vi "Bingo Lose.vi"() -> ()   [LabVIEW 2020]
uses:
  <vilib>/regexp/Match Regular Expression.xnode
panel:
  out "Losing Board":cluster{i32, bool}[][](array[cluster])
  out "x*y":i32
  out "Picks":string
  in  "Input":string="46,12,57,37,14,78,31,71,87,52,64,97,10,35,54,36,27,84,80,94,99,22,0,11,30,44,86,59,66,7,90,21,51,53,92,8,76,41,39,77,42,88,29,24,60,17,68,13,79,67,50,82,25,61,20,16,6,3,81,19,85,9,28,56,75,96,2,26,1,62,33,63,32,73,18,48,43,65,98,5,91,69,47,4,38,23,49,34,55,83,93,45,72,95,40,15,58,74,70,89\n\n37 72 60 35 89\n32 49  4 77 82\n30 26 27 63 88\n29 43 16 34 58\n48 33 96 79 94\n\n41 94 77 43 87\n 2 17 82 96 25\n95 49 32 12  9\n59 33 67 71 64\n88 54 93 85 30\n\n78 84 73 64 81\n 6 66 54 21 15\n72 88 69  5 93\n11 96 38 95 44\n13 41 94 55 48\n\n 5 14  2 82 33\n56 26  0 84 92\n 8 95 24 54 25\n68 67 15 85 47\n20 91 36 13 88\n\n39 26 33 65 32\n78 72 80 51  0\n35 64 60 18 31\n93 59 83 54 74\n86  5  9 98 69\n\n 0  8 20 18 70\n 5 29 65 21 57\n68 61 83 63 51\n91 73 77 75 80\n35 62 16 32 10\n\n51 78 58 67 93\n50 14 99  5 31\n 6 21 48 30 83\n22 33 23  1 34\n 2 72 57 54 42\n\n15 68  4 24 49\n12  9 74 88 51\n91 19 50 76 75\n80 84 23 17 53\n67 42 22 85 36\n\n41 78 11 69  9\n90 25 98 65 77\n97 53 37 84 89\n58 63  5 55  1\n24 10 74 20 82\n\n42 19 95 89 49\n61 31 50 76  3\n34 47 32 69 86\n78 68 99 11 91\n55 12 73 45 23\n\n24 53 95 64 14\n40 29 71 57 97\n62 70 25 22  2\n88 68 33 82 59\n72 38 76 78 43\n\n73 36 84 90 40\n16  4 57  9 29\n38 97 46 51 83\n86 88 99 44 32\n54 49 37 43 62\n\n18 66 17 49 27\n24 93 91 87 72\n54 37 77 43 10\n88 80 60 15 79\n47 68 12  2 69\n\n 9 23 13 57 68\n38 97 63 88 98\n96 62 65 82 58\n61 83 29 47 40\n21 86 20 16 56\n\n27 90 37 97 52\n14 96 76 21 79\n 0 43 63 81 56\n42 62 23 55 74\n45 72 77 44 47\n\n 8 78 63 24 87\n 9 23 12 17 68\n36 83 45 61 50\n84 77 18 86 37\n31 26 19 49 94\n\n72 84 59 48 40\n92 98 35  1 80\n83 15 85 63 39\n 2 64 58 13 20\n29 88 60 12 74\n\n21 94 52  6  4\n89 70 39 23 64\n96 87 31 54 14\n88 35 83 13 56\n84 10 98 48 68\n\n70 33 48 21 37\n91 95 65 38 77\n92 14 26 96 60\n12  6 73 13 81\n54 55  2 45 80\n\n60 11 67 95 28\n 5 32  0 71 12\n47 78 13 54 43\n49 89 82 66 77\n26 53 19 79  3\n\n81  9 53 72 29\n56 35 60 44 45\n42 94 96 88 64\n15 92  4  6 14\n97 11 17 61 63\n\n24 43 33  9 34\n36 28 69 35  7\n47  4 14 82 38\n11  1 52  0 49\n93 87 98 41  5\n\n37 79 99 34 77\n38 26 25 95 70\n28 78 40 33 86\n41 57 96 10 24\n 9 74 72 50 81\n\n18 96 52 29 61\n38 90  1 48 51\n78 11 27 55 97\n33 21 87 93 67\n79 46 94 45  2\n\n27 63  6 90 10\n 3 60 24  5 89\n78 72 76 54  8\n33 22 87 51 58\n 4 37 64 91 43\n\n63 73 87 80 89\n29 14 95 48  3\n71 55 69  9 67\n30 99 19  2 86\n26 72 88 85 37\n\n12 57 81 78 40\n35  4 55 15 39\n33 45 25 60 70\n86 79 88 52  3\n90 20 28 59 85\n\n92 51 98 47 99\n41 78 65  4 46\n19 87 39 89 17\n12 23 36 29 44\n 6 82 71 16 37\n\n 8 34 81 67 80\n83 92 13 11 41\n39 89 93 49 43\n20 69  3 74 76\n44 72 68 70 45\n\n66 39 94 98 28\n72  4 25 77 76\n56 41 84 59 40\n36 87 18 44 73\n29 45 79 55 95\n\n45 91  2 92 16\n21 47 86 81 56\n31 11 62  5 95\n39  1 30 65 33\n42 60 17 18 83\n\n86 11 77 30 43\n51 88 73 98 94\n72 63 38 56 10\n57 92 49  7 41\n79 75 34 23 54\n\n56 95  3 43 65\n39 62 93 19 27\n61 41 99 96 52\n 4 92 77 98 70\n16 54 11 17 57\n\n 6 63 10 71 58\n64 70 50 92  0\n 7 14 99 45 26\n78 17 44 46 73\n77 38 62 53 37\n\n31 82 67 55 27\n57 58 84  6 15\n14 41 49  8 85\n12 32 91 42 19\n23  1 87 54 29\n\n54 60 43 26  4\n78 17 28 67  5\n87 93 90 71 22\n13 30 16 21 85\n55 74 52  1 29\n\n50 16 70 32 33\n 6 94 52 66 22\n97 64 98 72 39\n27 69 99 34 26\n36 91 37 21 14\n\n 7 97 64 28 18\n85 80 14 37 34\n72  1 22 58 73\n53  3 68 17  0\n29 44 56 95 32\n\n30 66 93 24 92\n48 80 79 86 27\n89 13 62 94 81\n70 65 61  8 54\n96 97 20 90 34\n\n87 76  4  7 43\n92 55 80 25 62\n79  6 88 35 30\n10 32  5 45 17\n36 27 33 68 63\n\n72 69 27 88 41\n34 53 42 84  3\n58 18 22 66 65\n 9 47 85 12 62\n73 90 91 57 33\n\n67 16 50 58 52\n68 70 84 98 69\n 4 72  9 64  0\n93 97 39 26  5\n 3 37 79  7 82\n\n61 57 88 54 70\n77  8 94 81 63\n39 48 18 13 10\n55 23 27  4 73\n 3  5 64  0 96\n\n62 27  0 52 19\n28 57 83 25 41\n 5 59 24 33 80\n37 85  2 86 43\n22 94 50  8 20\n\n54 32 34 47 87\n71 22 43 85 24\n11 68 58 36 46\n35 56 61 67 18\n70 23 72  5 59\n\n 3 96 41 45 32\n68  2 56 28 24\n87 38 40 75 26\n53 64 73 80 81\n54 88 20  6 18\n\n64 55 51 96 47\n59 35 49 67 71\n36 91 61 76 68\n 6 94 20  8 27\n60 88 45  7 82\n\n87 94 51 91  1\n96 60 28 97 37\n26 27 74 53 35\n88 89 11 77  8\n73 47 18 59  6\n\n46 50 19 36 83\n69 28  4 44 70\n45 20 63 27  1\n53 38  9 47 67\n91 31 79 73 86\n\n45  3 98 91 60\n40  7 78 34 83\n52 73 59 13  4\n38 15 82 86 79\n42 11 17 20 62\n\n65 86 38 20 72\n78 45 73 74 25\n62 42 24 75  3\n81  8 35 50 51\n44 11 94 85 57\n\n13 86 55 65 96\n53 18 43 76 20\n41 14 32 52 38\n90 59 80 68  7\n 2 23 92 39 50\n\n96 62 85 24 14\n37  5 11 91 45\n61 28 23 34 77\n43 48 20  0 21\n10 35  2 26 97\n\n89  5 40 34 84\n90  6 72 68 10\n13 64 71 31 76\n53 60  9 92 62\n69 98  8 50  3\n\n17 86 10 75 79\n67 94 78 40 56\n11 85 82 50 46\n53 39 22  9 61\n59 73 72 33 45\n\n65 22 18 96 95\n55 86 67 52 69\n10  2 60 83 98\n43 61 87 88 66\n41 24  8 84 33\n\n31 53 98 70 91\n33 34 48 83  9\n40 39 29 71 65\n69 10 62 30  4\n52 21 11 93 75\n\n 8 94 53 85 89\n13 84 58 59 29\n97  7 21 25 96\n45 54 34 22 63\n37 17 49 68 67\n\n86 87 84 24 10\n82 32 36 59 50\n 8 62 79 71 43\n49 23 85 69 58\n21 66 42 25 56\n\n65 88 43 25 19\n26 36 63  5  6\n37 54 75  1 38\n95 46 83 66 28\n 4 90 80 99 85\n\n78 83  7 77 34\n27 92 93 96 82\n40 95 52 32 43\n17 28 69 41 85\n21 65 39 58 19\n\n11 84 28 90 36\n74  4 62  5 46\n22  8 45 40 98\n12  6 30  9 82\n37  2 53 29 41\n\n17 65 31 86 57\n73 16 24 67 53\n60 93 88 45 26\n14 80 94  7 44\n55 78 49  8 82\n\n95 38 81 25 76\n29 13 83 47 12\n17 69  4 43 28\n63 84 39 52 34\n 1 97 41 88  8\n\n70 40 16 83  3\n15 49 20 74 48\n71 30 21 28 84\n29 10 97  1 18\n57 50 63 35 69\n\n40 13 67  9 41\n71 76  8 54 24\n15 97 92 49 96\n61 34 23 81 31\n11 38 48 37 86\n\n77 36 32 75  7\n38 18 84 26  2\n19 13 99 83 20\n35 51 74  6 27\n71 48 15 66 69\n\n91 57 41  3 99\n74 55 81 77 43\n36 52 47 49 45\n85 65  5 38 50\n90 68 70 16  0\n\n 1 90 28 86 27\n73 36 67 11 14\n71 31 10 65 55\n78 21 16 69 12\n87 24 33 83 68\n\n90 17 10 84 45\n 5 68 69 27 92\n 6 63 98  3 46\n94 48 59 34 43\n39 88 12 33 73\n\n12 31 33 98 63\n65 51 94 83 92\n41 38 84 91 66\n47 28 76 54  3\n48 36 11 13 27\n\n51 84 96 16  8\n64 26 74 30 48\n29 41 68 97 87\n 9 38  1 15 39\n98  3 45 53 14\n\n53 70 90 95 86\n35 22 85 45 66\n93  0 83 30 88\n64 57 68 36  3\n 5 51 19 20 89\n\n 9 36 69 46 44\n37  7 99 57 45\n79 10 86 58 30\n49 98 52 90 27\n14 51 88 60 81\n\n73 97 91 19 48\n76 43 18 83 67\n62  9 11 82 55\n24 17 33 53 22\n75  8 56  1 21\n\n27 97 53  0 89\n30 70  3 80 54\n56 93 40 64 35\n46 82  1 44 65\n 6 59 45 32 34\n\n87 58 73 45 69\n24 49 89 71 83\n94  6 53 68 50\n28 25 88 47  0\n36 13 31 18 55\n\n52 63 37 66  9\n34 77 57  6 55\n85 80 97 78 74\n95 75 67 96 29\n22 73 92 69 47\n\n79 97 80 36 73\n38 77 35 32 53\n 2 37 29  6 89\n78 91 15 47 34\n11 52 64 84  0\n\n69 30 21 99 46\n72  4 15 25 42\n67 98 81 91 63\n70 20 57 65 14\n 0 78 19  8 87\n\n20  4 98 33 85\n76 17 94 65 35\n95 69 72 52 71\n23 25 50 38 27\n43 49 96 53 99\n\n16 27 34 65 36\n10 40 84 60 82\n80  2 54 67 70\n52 94 79 17 56\n 5 14 77 91 88\n\n32 90 50 66 39\n30 16 14 20 10\n 4 42 88 59 12\n75 84 54 51 48\n33 24 13 89 43\n\n78 42 34 65 51\n75 72  3 99 61\n15 50 59  8 89\n71 18  9 54 53\n43 39 97 56 19\n\n50 43 83  4 30\n89 97 58 35 39\n11 24 61 41 25\n87 99 93 15 34\n31 57  3 45 44\n\n70 21 63 24 38\n34 23 88  7 51\n43 18 76 46 49\n60 78 47  8 12\n11 66 98 25 74\n\n30 17 23 10 92\n12 85 69 81 91\n47 80 28 29 58\n73 44 77 50 32\n76 54 78 75 60\n\n71 53 86 48 98\n90 37 79  8 56\n99 42 97 36 15\n31 85 34 10 40\n43 89 57 72 51\n\n48  0 65 55 90\n45 76 69 97  4\n42 52 46 77 56\n64 62 68 35 72\n71 10 27 30 16\n\n41 69 63 88 57\n25 56 23 78 80\n 8 92 59 66 97\n48 61 77 15 14\n87 47 91 12 71\n\n51 46 15  2 49\n48 33 23 16  4\n80 41 43 59 83\n62 13 20 63 85\n99 30  7 87  8\n\n69 80 96 43 47\n61 75 45 62 15\n32 22 91 83 58\n82 13 50 52  8\n89 20 63 73 14\n\n40  2 96 52 73\n25 27 26 43 34\n60 38 80 78  5\n83 63 48 10 66\n97 46 53 74 86\n\n46  7  0 69 15\n79 19 85 27 73\n63 45  5 49 54\n93 29 84 28 66\n72 23 99  8 33\n\n20 72 85 99 49\n69  0 10 52 23\n88 56 28 67 21\n16 91 83 54 81\n14 73 32 30 59\n\n31 52 63 12  3\n96 20 82  6 89\n55 38  8 95 40\n 5 60 84 81 75\n51 14 65 27 61\n\n46 93  1 47 76\n 8 98  7 16 63\n44 78 17 14 92\n42 62 20 12 68\n56  3 74  6 21\n\n 8 94 11 40 44\n43 92 78 91 18\n75 80 12 54 26\n67  9 45 22 21\n86  1 90 36 30\n\n21 19 83 90  8\n50 28 45 65 75\n59 88 25 29 70\n58 23  0 95 49\n36 68 76 78 66\n\n77 28 43 56 97\n73 71  8 72 46\n23 25 70 69 41\n90 17 34 67 48\n32 75 81 63 21"
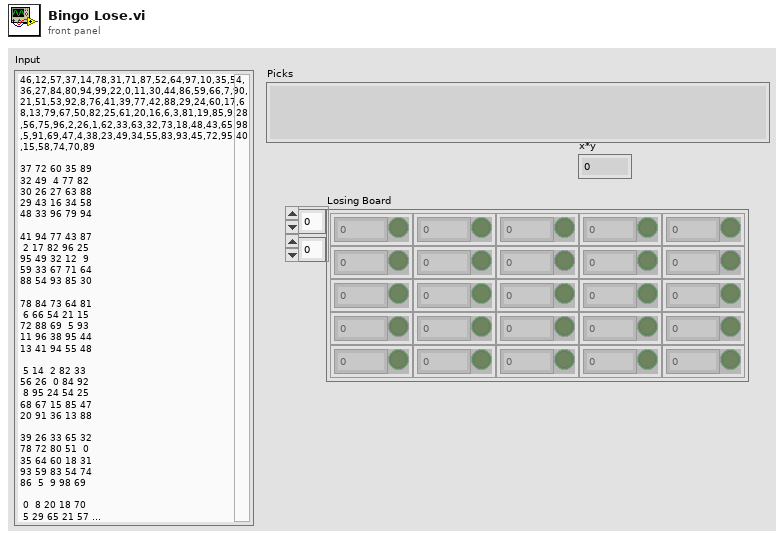
[diagram p1: front panel]
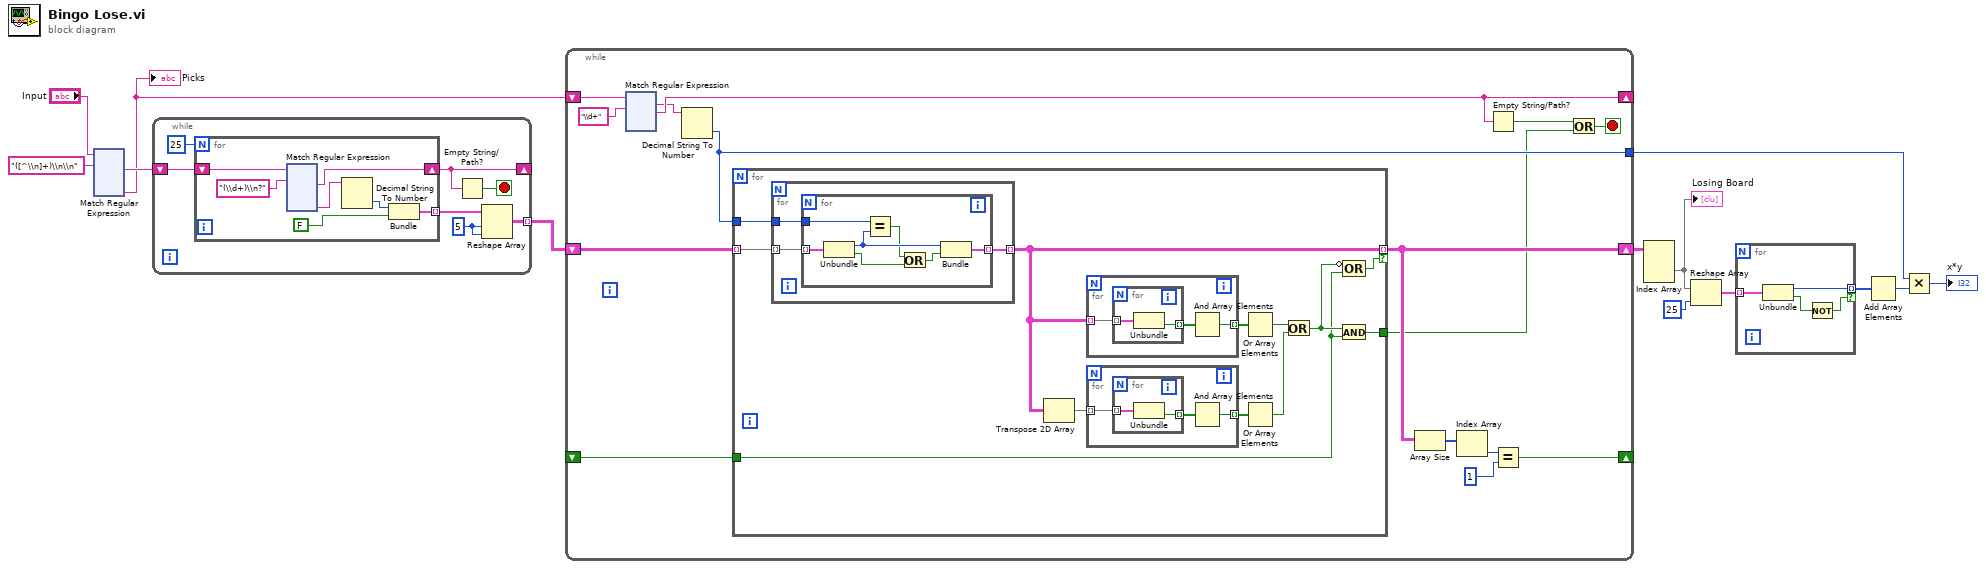
[diagram p0: block diagram]
diagram:
  n1 = xnode "Match Regular Expression"("input string"="Input", "regular expression"="([^\\n]+)\\n\\n") -> ("after match"=w11:string, "submatch 1"=w10:string)  [unwired: 4 in, 4 out]
  "Picks" <- w10
  n2 = while {
    shift-right: [w19] -> _
    shift-left: w11 -> [w20]
    tunnel: [w14] -> w9 mode=indexing
    stop <- w18 stop-if-true
    w15 = 5 ("dimension size")
    n3 = for {
      N: 25 -> [_]
      shift-right: [w25] -> w19
      shift-left: w20 -> [w27]
      tunnel: [w23] -> w16 mode=indexing
      n4 = xnode "Match Regular Expression"("input string"=w27, "regular expression"="(\\d+)\\n?") -> ("after match"=w25:string, "submatch 1"=w22:string)  [unwired: 4 in, 4 out]
      n5 = Decimal String To Number(string=w22) -> (number=w21:i32)  [unwired: 2 in, 1 out]
      n6 = Bundle(w21, FALSE) -> (w23:cluster{i32, bool})  [unwired: 1 in]
    }
    n7 = Empty String/Path?(string/path=w19) -> (empty?=w18:bool)
    n8 = Reshape Array(w16, w15, w15) -> (w14:cluster{i32, bool}[][])
  }
  n9 = while {
    shift-right: [w155] -> _
    shift-left: w10 -> [w158]
    shift-right: [w150] -> w2
    shift-left: w9 -> [w153]
    tunnel: [w151] -> w4
    shift-right: [w146] -> _
    shift-left: _ -> [w145]
    stop <- w152 stop-if-true
    n10 = xnode "Match Regular Expression"("input string"=w158, "regular expression"="\\d+") -> ("whole match"=w154:string, "after match"=w155:string)  [unwired: 4 in, 3 out]
    n11 = Decimal String To Number(string=w154) -> (number=w151:i32)  [unwired: 2 in, 1 out]
    n12 = for {
      tunnel: w153 -> [w284] mode=indexing
      tunnel: w151 -> [w283]
      tunnel: [w277] -> w150 mode=indexing if=w276
      tunnel: w145 -> [w274]
      tunnel: [w273] -> w144
      n13 = for {
        tunnel: w284 -> [w297] mode=indexing
        tunnel: w283 -> [w296]
        tunnel: [w295] -> w277 mode=indexing
        n14 = for {
          tunnel: w297 -> [w304] mode=indexing
          tunnel: w296 -> [w303]
          tunnel: [w298] -> w295 mode=indexing
          n15 = Unbundle(w304) -> (w302:i32, w301:bool)
          n16 = Equal?(x=w303, y=w302) -> (x = y?=w300:bool)
          n17 = Or(x=w300, y=w301) -> (x .or. y?=w299:bool)
          n18 = Bundle(w302, w299) -> (w298:cluster{i32, bool})  [unwired: 1 in]
        }
      }
      n19 = Transpose 2D Array(2D array=w277) -> (transposed array=w280:cluster{i32, bool}[][])
      n20 = for {
        tunnel: w277 -> [w292] mode=indexing
        tunnel: [w290] -> w282 mode=indexing
        n21 = for {
          tunnel: w292 -> [w294] mode=indexing
          tunnel: [w293] -> w291 mode=indexing
          n22 = Unbundle(w294) -> (w293:bool)  [unwired: 1 out]
        }
        n23 = And Array Elements(Boolean array=w291) -> (logical AND=w290:bool)
      }
      n24 = for {
        tunnel: w280 -> [w287] mode=indexing
        tunnel: [w285] -> w281 mode=indexing
        n25 = for {
          tunnel: w287 -> [w289] mode=indexing
          tunnel: [w288] -> w286 mode=indexing
          n26 = Unbundle(w289) -> (w288:bool)  [unwired: 1 out]
        }
        n27 = And Array Elements(Boolean array=w286) -> (logical AND=w285:bool)
      }
      n28 = Or Array Elements(Boolean array=w282) -> (logical OR=w279:bool)
      n29 = Or Array Elements(Boolean array=w281) -> (logical OR=w278:bool)
      n30 = Or(x=w279, y=w278) -> (x .or. y?=w275:bool)
      n31 = And(x=w275, y=w274) -> (x .and. y?=w273:bool)
      n32 = Compound Arithmetic op=OR(invert w275, w274) -> (w276:bool)
    }
    n33 = Array Size(array=w150) -> (size(s)=w149:i32[])
    n34 = Index Array(array=w149) -> (element=w148:i32)  [unwired: 1 in]
    n35 = Empty String/Path?(string/path=w155) -> (empty?=w156:bool)
    n36 = Equal?(x=w148, y=1) -> (x = y?=w146:bool)
    n37 = Or(x=w156, y=w144) -> (x .or. y?=w152:bool)
  }
  n38 = Index Array(array=w2) -> (element=w1:cluster{i32, bool}[][])  [unwired: 3 in]
  "Losing Board" <- w1
  n39 = Reshape Array(w1, 25 ("dimension size")) -> (w7:cluster{i32, bool}[])
  n40 = for {
    tunnel: w7 -> [w308] mode=indexing
    tunnel: [w307] -> w6 mode=indexing if=w305
    n41 = Unbundle(w308) -> (w307:i32, w306:bool)
    n42 = Not(x=w306) -> (.not. x?=w305:bool)
  }
  n43 = Add Array Elements(numeric array=w6) -> (sum=w5:i32)
  n44 = Multiply(x=w4, y=w5) -> (x*y=→"x*y":i32)
